vi "Setup SSHAskPass.vi"(4 "password":string, 6 "password specified?":bool, 8 "error in (no error)":errorcluster, 11 "OpenSSH Client in":refnum<class "OpenSSH Client.lvclass">) -> (0 "error out":errorcluster, 1 "SSH PW Pipe":string, 2 "environment variables":cluster{"name":string, "value":string}[](array[cluster]), 3 "OpenSSH Client out":refnum<class "OpenSSH Client.lvclass">)   [LabVIEW 2020, in "NI_SSH.lvlib" / "OpenSSH Client.lvclass"]
uses:
  <vilib>/net/SSH/Client/OpenSSH/OpenSSH Client.lvclass
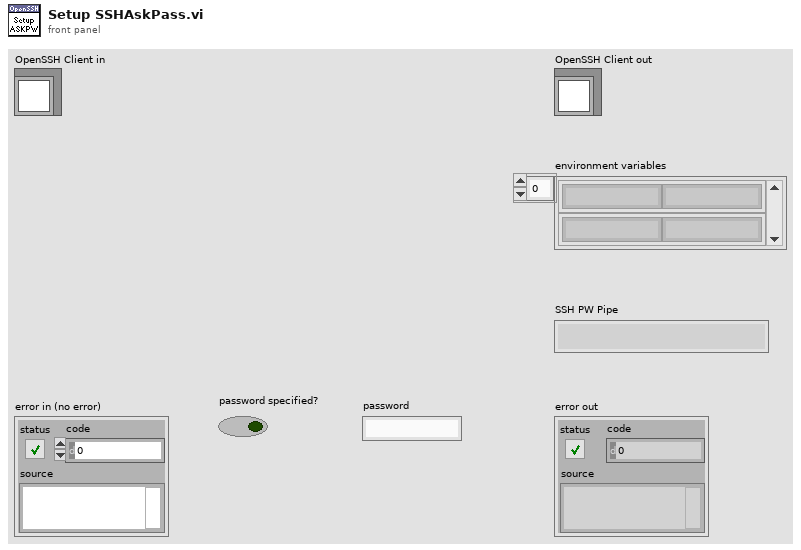
[diagram p1: front panel]
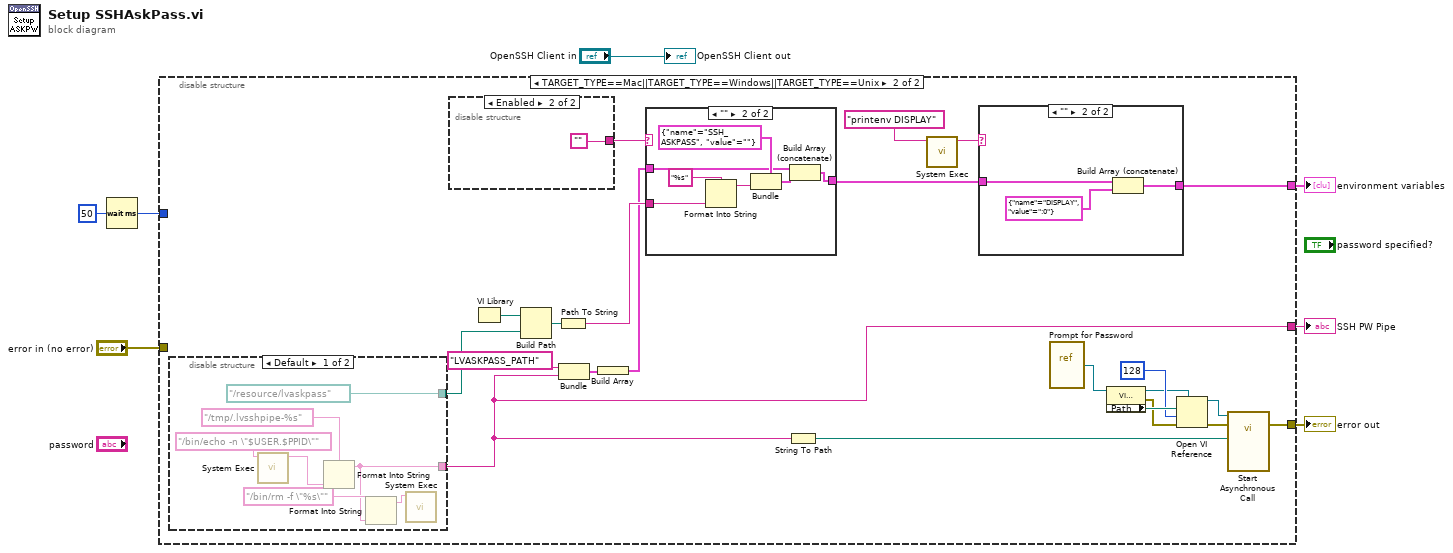
[diagram p0: block diagram]
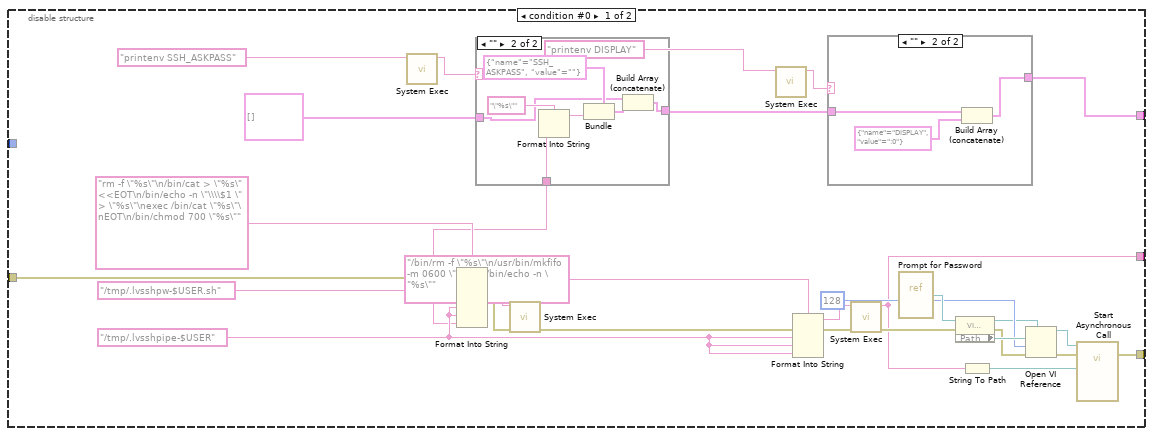
[diagram p2: hidden frame]
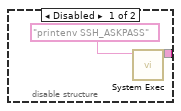
[diagram p5: hidden frame]
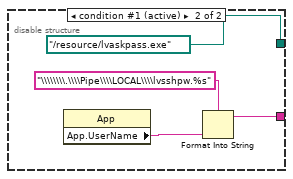
[diagram p6: hidden frame]
diagram:
  n1 = Wait (ms)(milliseconds to wait=u32 50) -> (millisecond timer value=w1:u32)
  n2 = disable-structure "Conditional Disable Structure" shown="TARGET_TYPE==Mac||TARGET_TYPE==Windows||TARGET_TYPE==Unix" {
    disable-tunnel: "error in (no error)" -> [w30 _]
    disable-tunnel: [w22 w63] -> w6
    disable-tunnel: [w18 w49] -> w5
    disable-tunnel: [w15 w61] -> w3
    disable-tunnel: w1 -> [_ _]
    frame condition #0 {
      w19 = "/tmp/.lvsshpipe-$USER"
      w8 = "/tmp/.lvsshpw-$USER.sh"
      n3 = call <vilib>:"System Exec.vi"("command line"="printenv SSH_ASKPASS") -> ("standard output"=w13:string)  [unwired: 7 in, 3 out]
      n4 = Format Into String(format string="rm -f \"%s\"\n/bin/cat > \"%s\" <<EOT\n/bin/echo -n \"\\\\$1 \" > \"%s\"\nexec /bin/cat \"%s\"\nEOT\n/bin/chmod 700 \"%s\"" ("command line"), error in=w30, w8, w8, w19, w19, w8) -> (resulting string=w34:string, error out=w31:errorcluster)  [unwired: 1 in]
      n5 = case shown="\"\"" w13 {
        tunnel: w8 -> [_ w44]
        tunnel: [w40 w41] -> w12
        tunnel: cluster{"name":string, "value":string}[] [] ("appended array") -> [w40 w42]
        frame Default {
        }
        frame "" {
          n6 = Format Into String(format string="\"%s\"" ("prefix string"), w44) -> (resulting string=w47:string)  [unwired: 2 in, 1 out]
          n7 = Bundle(cluster=cluster{"name":string, "value":string} {"name"="SSH_ASKPASS", "value"=""} ("environment variable"), "value"=w47) -> (w43:cluster{"name":string, "value":string})  [unwired: 1 in]
          n8 = Build Array (concatenate)(w42, w43) -> (w41:cluster{"name":string, "value":string}[])
        }
      }
      n9 = call <vilib>:"System Exec.vi"("error in (no error)"=w31, "command line"=w34) -> ("error out"=w17:errorcluster)  [unwired: 6 in, 3 out]
      n10 = call <vilib>:"System Exec.vi"("command line"="printenv DISPLAY") -> ("standard output"=w9:string)  [unwired: 7 in, 3 out]
      n11 = Format Into String(format string="/bin/rm -f \"%s\"\n/usr/bin/mkfifo -m 0600 \"%s\"\n/bin/echo -n \"%s\"" ("command line"), error in=w17, w19, w19, w19) -> (resulting string=w32:string, error out=w16:errorcluster)  [unwired: 1 in]
      n12 = case shown="\"\"" w9 {
        tunnel: [w36 w38] -> w15
        tunnel: w12 -> [w36 w37]
        frame Default {
        }
        frame "" {
          n13 = Build Array (concatenate)(w37, cluster{"name":string, "value":string} {"name"="DISPLAY", "value"=":0"} ("environment variable")) -> (w38:cluster{"name":string, "value":string}[])
        }
      }
      n14 = call <vilib>:"System Exec.vi"("error in (no error)"=w16, "command line"=w32) -> ("error out"=w25:errorcluster, "standard output"=w18:string)  [unwired: 6 in, 2 out]
      n15 = vi-ref <vilib>:"Prompt for Password.vi"() -> (w29:refnum<vi>)
      n16 = property on="Property Node" class="VI (strict)"(reference=w29, error in=w25) -> (reference out=w20:refnum<vi>, error out=w24:errorcluster, "Path"=w28:path)
      n17 = String To Path(string=w18) -> (path=w21:path)
      n18 = Open VI Reference(type specifier VI Refnum (for type only)=w20, vi path=w28, options=128, error in (no error)=w24) -> (vi reference=w26:refnum<vi>, error out=w23:errorcluster)  [unwired: 2 in]
      n19 = call-by-ref "Start Asynchronous Call"(reference=w26, error in=w23, "Pipe Path"=w21) -> (error out=w22:errorcluster)  [unwired: 11 in, 1 out]
    }
    frame condition #1 (active) {
      n20 = disable-structure shown="Default" {
        disable-tunnel: [path "../resource/lvaskpass" ("name or relative path") path "../resource/lvaskpass.exe" ("name or relative path")] -> w50
        disable-tunnel: [w74 w80] -> w49
        frame condition #0 {
          n21 = call <vilib>:"System Exec.vi"("command line"="/bin/echo -n \"$USER.$PPID\"") -> ("standard output"=w76:string)  [unwired: 7 in, 3 out]
          n22 = Format Into String(format string="/tmp/.lvsshpipe-%s", w76) -> (resulting string=w74:string)  [unwired: 2 in, 1 out]
          n23 = Format Into String(format string="/bin/rm -f \"%s\"", w74) -> (resulting string=w73:string)  [unwired: 2 in, 1 out]
          n24 = call <vilib>:"System Exec.vi"("command line"=w73) -> ()  [unwired: 7 in, 4 out]
        }
        frame condition #1 (active) {
          n25 = property class="App"() -> ("App.UserName"=w83:string)  [unwired: 2 in, 2 out]
          n26 = Format Into String(format string="\\\\\\\\.\\\\Pipe\\\\LOCAL\\\\lvsshpw.%s", w83) -> (resulting string=w80:string)  [unwired: 2 in, 1 out]
        }
      }
      n27 = disable-structure shown="Enabled" {
        disable-tunnel: [w70 ""] -> w60
        frame Disabled {
          n28 = call <vilib>:"System Exec.vi"("command line"="printenv SSH_ASKPASS") -> ("standard output"=w70:string)  [unwired: 7 in, 3 out]
        }
        frame Enabled {
        }
      }
      n29 = VI Library() -> (path=w56:path)
      n30 = Build Path(base path=w56, name or relative path=w50) -> (appended path=w55:path)
      n31 = Path To String(path=w55) -> (string=w54:string)
      n32 = Bundle("LVASKPASS_PATH", w49) -> (w52:cluster{string, string})  [unwired: 1 in]
      n33 = Build Array(w52) -> (w51:cluster{string, string}[])
      n34 = case shown="\"\"" w60 {
        tunnel: w54 -> [_ w92]
        tunnel: [w88 w89] -> w59
        tunnel: w51 -> [w88 w90]
        frame Default {
        }
        frame "" {
          n35 = Format Into String(format string="%s" ("prefix string"), w92) -> (resulting string=w95:string)  [unwired: 2 in, 1 out]
          n36 = Bundle(cluster=cluster{"name":string, "value":string} {"name"="SSH_ASKPASS", "value"=""} ("environment variable"), "value"=w95) -> (w91:cluster{"name":string, "value":string})  [unwired: 1 in]
          n37 = Build Array (concatenate)(w90, w91) -> (w89:cluster{"name":string, "value":string}[])
        }
      }
      n38 = String To Path(string=w49) -> (path=w48:path)
      n39 = call <vilib>:"System Exec.vi"("command line"="printenv DISPLAY") -> ("standard output"=w57:string)  [unwired: 7 in, 3 out]
      n40 = case shown="\"\"" w57 {
        tunnel: [w84 w86] -> w61
        tunnel: w59 -> [w84 w85]
        frame Default {
        }
        frame "" {
          n41 = Build Array (concatenate)(w85, cluster{"name":string, "value":string} {"name"="DISPLAY", "value"=":0"} ("environment variable")) -> (w86:cluster{"name":string, "value":string}[])
        }
      }
      n42 = vi-ref <vilib>:"Prompt for Password.vi"() -> (w69:refnum<vi>)
      n43 = property on="Property Node" class="VI (strict)"(reference=w69) -> (reference out=w62:refnum<vi>, error out=w65:errorcluster, "Path"=w68:path)  [unwired: 1 in]
      n44 = Open VI Reference(type specifier VI Refnum (for type only)=w62, vi path=w68, options=128, error in (no error)=w65) -> (vi reference=w66:refnum<vi>, error out=w64:errorcluster)  [unwired: 2 in]
      n45 = call-by-ref "Start Asynchronous Call"(reference=w66, error in=w64, "Pipe Path"=w48) -> (error out=w63:errorcluster)  [unwired: 11 in, 1 out]
    }
  }
  "error out" <- w6
  "SSH PW Pipe" <- w5
  "environment variables" <- w3
  "OpenSSH Client out" <- "OpenSSH Client in"
